vi "AMZ_S3_APIHLP_Parse AccessControlPolicy.vi"(8 "error in (no error)":errorcluster, 10 "Response body":string) -> (0 "error out":errorcluster, 3 "AccessControlPolicy":T1)   [LabVIEW 2015, in "LV Interface for Amazon S3.lvlib"]
uses:
  LV Interface for Amazon S3.lvlib
  Typedefs/AMZ_S3_API_AccessControlPolicy.ctl
  Typedefs/AMZ_S3_API_Owner.ctl
  Typedefs/AMZ_S3_API_Bucket ACL Permission.ctl
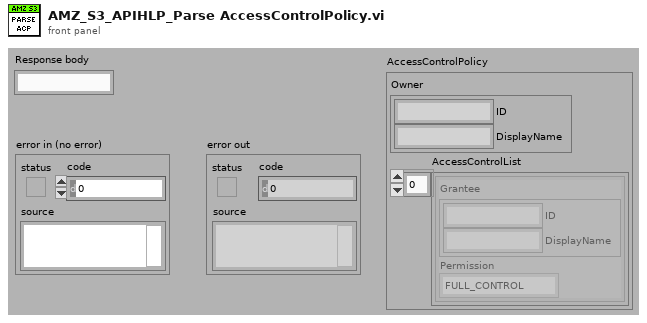
[diagram p1: front panel]
types:
  T1 = typedef "LV Interface for Amazon S3.lvlib/AMZ_S3_API_AccessControlPolicy.ctl" = cluster{"Owner":T2, "AccessControlList":cluster{"Grantee":T2, "Permission":T3}[]}
  T2 = typedef "LV Interface for Amazon S3.lvlib/AMZ_S3_API_Owner.ctl" = cluster{"ID":string, "DisplayName":string}
  T3 = typedef "LV Interface for Amazon S3.lvlib/AMZ_S3_API_Bucket ACL Permission.ctl" = enum16{"FULL_CONTROL", "WRITE", "WRITE_ACP", "READ", "READ_ACP"}
  T4 = cluster{cluster{"Value":string, "Value":string}, "Permission":T3}
  T5 = cluster{cluster{"Value":string, "Value":string}, "Permission":T3}[]
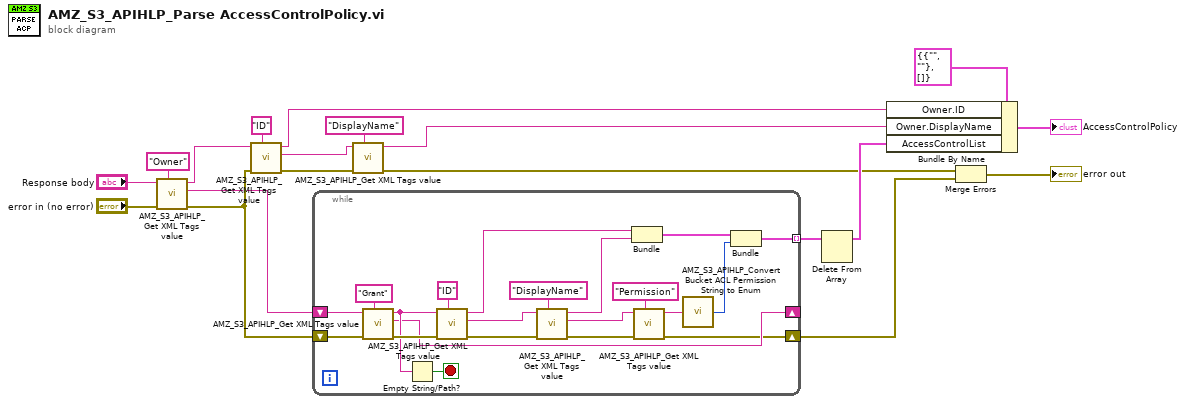
[diagram p0: block diagram]
diagram:
  n1 = call "AMZ_S3_APIHLP_Get XML Tags value.vi"("Tag name"="Owner", "error in (no error)"="error in (no error)", "XML String in"="Response body") -> ("error out"=w8:errorcluster, "Remaining string"=w7:string, "Value"=w16:string)  [unwired: 6 in]
  n2 = call "AMZ_S3_APIHLP_Get XML Tags value.vi"("Tag name"="ID", "error in (no error)"=w8, "XML String in"=w16) -> ("error out"=w14:errorcluster, "Remaining string"=w12:string, "Value"=w10:string)  [unwired: 6 in]
  n3 = while {
    shift-right: [w30] -> _
    shift-left: w7 -> [w39]
    tunnel: [w21] -> w6 mode=indexing
    shift-right: [w20] -> w2
    shift-left: w8 -> [w40]
    stop <- w37 stop-if-true
    n4 = call "AMZ_S3_APIHLP_Get XML Tags value.vi"("Tag name"="Grant", "error in (no error)"=w40, "XML String in"=w39) -> ("error out"=w36:errorcluster, "Remaining string"=w30:string, "Value"=w35:string)  [unwired: 6 in]
    n5 = Empty String/Path?(string/path=w35) -> (empty?=w37:bool)
    n6 = call "AMZ_S3_APIHLP_Get XML Tags value.vi"("Tag name"="ID", "error in (no error)"=w36, "XML String in"=w35) -> ("error out"=w32:errorcluster, "Remaining string"=w31:string, "Value"=w25:string)  [unwired: 6 in]
    n7 = call "AMZ_S3_APIHLP_Get XML Tags value.vi"("Tag name"="DisplayName", "error in (no error)"=w32, "XML String in"=w31) -> ("error out"=w29:errorcluster, "Remaining string"=w28:string, "Value"=w24:string)  [unwired: 6 in]
    n8 = Bundle("Value"=w25, "Value"=w24) -> (w23:cluster{"Value":string, "Value":string})  [unwired: 1 in]
    n9 = call "AMZ_S3_APIHLP_Get XML Tags value.vi"("Tag name"="Permission", "error in (no error)"=w29, "XML String in"=w28) -> ("error out"=w20:errorcluster, "Value"=w26:string)  [unwired: 6 in, 1 out]
    n10 = call "AMZ_S3_APIHLP_Convert Bucket ACL Permission String to Enum.vi"("Permission String"=w26) -> ("Permission"=w22:T3)  [unwired: 4 in]
    n11 = Bundle(w23, "Permission"=w22) -> (w21:T4)  [unwired: 1 in]
  }
  n12 = call "AMZ_S3_APIHLP_Get XML Tags value.vi"("Tag name"="DisplayName", "error in (no error)"=w14, "XML String in"=w12) -> ("error out"=w3:errorcluster, "Value"=w9:string)  [unwired: 6 in, 1 out]
  n13 = Delete From Array(array=w6) -> (array with subset deleted=w5:T5)  [unwired: 2 in, 1 out]
  n14 = Bundle By Name(cluster=T1 {"Owner"={"ID"="", "DisplayName"=""}, "AccessControlList"=[]} ("AccessControlPolicy"), "Owner.ID"=w10, "Owner.DisplayName"=w9, "AccessControlList"=w5) -> (→"AccessControlPolicy":T1)
  n15 = Merge Errors(w3, w2) -> (→"error out":errorcluster)
